vi "TC-01-(Acquire)UpdateCVT.vi"(8 "error in (no error)":errorcluster, 11 "NI-TC-01 in":refnum<class "NI-TC-01.lvclass">) -> (0 "error out":errorcluster, 3 "NI-TC-01 out":refnum<class "NI-TC-01.lvclass">)   [LabVIEW 2020, in "NI-TC-01.lvclass"]
uses:
  NI-TC-01.lvclass
  NI-TC-01.lvclass/NI-TC-01.ctl
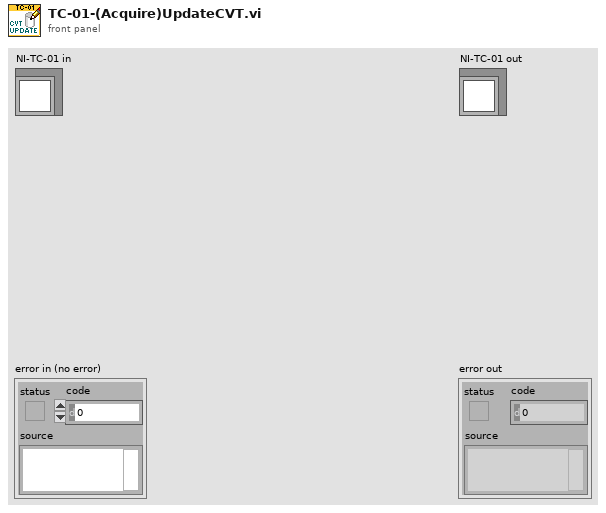
[diagram p1: front panel]
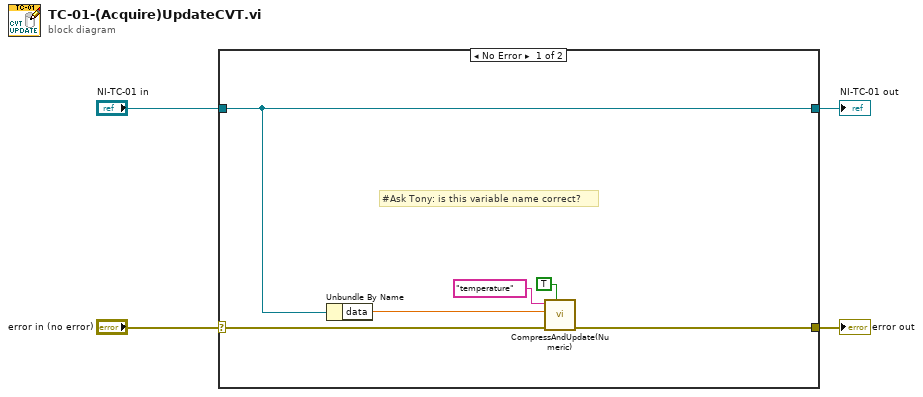
[diagram p0: block diagram]
diagram:
  n1 = case shown="No Error" "error in (no error)" {
    selector: "error in (no error)" -> [w9 w12]
    tunnel: [w8 w12] -> w3
    tunnel: [w7 w11] -> w1
    tunnel: "NI-TC-01 in" -> [w7 w11]
    frame No Error {
      # "#Ask Tony: is this variable name correct?"
      n2 = Unbundle By Name(w7) -> ("data"=w6:dbl)
      n3 = call "CompressAndUpdate(Numeric).vi"("force CVT update (false)"=TRUE, "error in"=w9, "Numeric"=w6, "command or variable name"="temperature") -> ("error out"=w8:errorcluster)  [unwired: 7 in]
    }
    frame Error {
    }
  }
  "error out" <- w3
  "NI-TC-01 out" <- w1
